vi "NKTP_API_UserEventExample.vi"() -> ()   [LabVIEW 2015]
doc: "This VI is a template that can be used when you want to make LabVIEW code that registers events from the NKTP driver as LabVIEW events in an event structure.\nPlease consult the \"NKTP_API_RegUserEvents.vi\" VI documentation for more information regarding using LabVIEW events with the NKTP driver."
uses:
  <instrlib>/NKTP_API/Public/Event/NKTP_API_RegisterDataType.ctl
  <instrlib>/NKTP_API/Private/NKTP_API_ParametersetType.ctl
  <instrlib>/NKTP_API/Public/Event/NKTP_API_DeviceStatusCallbackType.ctl
  <instrlib>/NKTP_API/Private/NKTP_API_DeviceCallbackStatusTypes.ctl
  <instrlib>/NKTP_API/Public/Event/NKTP_API_PortStatusCallbackType.ctl
  <instrlib>/NKTP_API/Private/NKTP_API_PortCallbackStatusTypes.ctl
  <instrlib>/NKTP_API/Public/Event/NKTP_API_RegisterStatusCallbackType.ctl
  <instrlib>/NKTP_API/Private/NKTP_API_RegisterCallbackStatusTypes.ctl
  <instrlib>/NKTP_API/Private/NKTP_API_RegisterDataTypes.ctl
  <instrlib>/NKTP_API/Private/NKTP_API_RegisterPriorityTypes.ctl
  <instrlib>/NKTP_API/NKTP_API.lvlib
panel:
  out "RegisterStatusCallbackData":T1={"portname"="", "devId"=0, "regId"=0, "status"=enum."RegSucces", "type"=enum."RegData_Array", "regDataLen"=0, "regData"=[]} {"regId" format="%.0x"}
  out "PortStatusCallbackData":T4={"portname"="", "status"=enum."PortStatusUnknown", "curScanAdr"=0, "maxScanAdr"=0, "foundType"=1}
  out "DeviceStatusCallbackData":T6
  in  "VISA Resource Name":refnum<visa-resource-name>
  out "RegisterData":T8
  out "error out":errorcluster
  in  "Close":bool
  in  "Open":bool
  in  "stop":bool
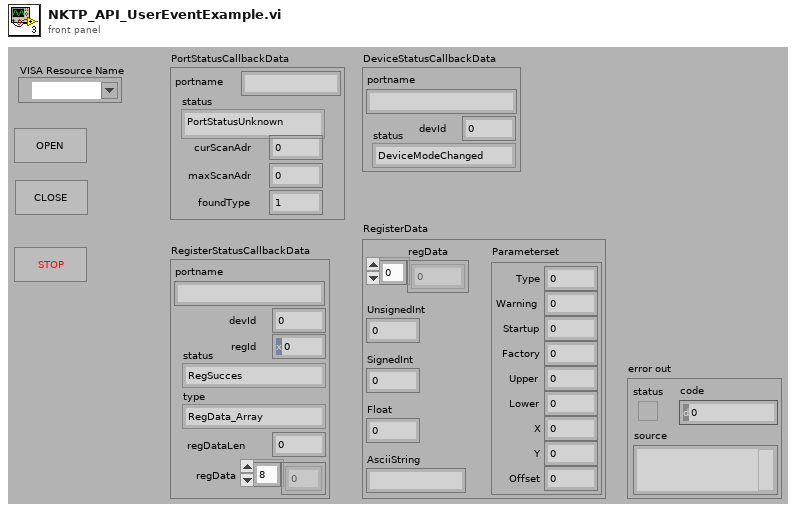
[diagram p1: front panel]
types:
  T1 = typedef "NKTP_API.lvlib/NKTP_API_RegisterStatusCallbackType.ctl" = cluster{"portname":string, "devId":u8, "regId":u8, "status":T2, "type":T3, "regDataLen":u8, "regData":u8[]}
  T2 = typedef "NKTP_API.lvlib/NKTP_API_RegisterCallbackStatusTypes.ctl" = enum8{"RegSucces", "RegBusy", "RegNacked", "RegCRCErr", "RegTimeout", "RegComError"}
  T3 = typedef "NKTP_API.lvlib/NKTP_API_RegisterDataTypes.ctl" = enum8{"RegData_Unknown", "RegData_Array", "RegData_U8", "RegData_S8", "RegData_U16", "RegData_S16", "RegData_U32", "RegData_S32", "RegData_F32", "RegData_U64", "RegData_S64", "RegData_F64", "RegData_Ascii", "RegData_Paramset"}
  T4 = typedef "NKTP_API.lvlib/NKTP_API_PortStatusCallbackType.ctl" = cluster{"portname":string, "status":T5, "curScanAdr":u8, "maxScanAdr":u8, "foundType":u16}
  T5 = typedef "NKTP_API.lvlib/NKTP_API_PortCallbackStatusTypes.ctl" = enum8{"PortStatusUnknown", "PortOpening", "PortOpened", "PortOpenFail", "PortScanStarted", "PortScanProgress", "PortScanDeviceFound", "PortScanEnded ", "PortClosing", "PortClosed", "PortReady"}
  T6 = typedef "NKTP_API.lvlib/NKTP_API_DeviceStatusCallbackType.ctl" = cluster{"portname":string, "devId":u8, "status":T7}
  T7 = typedef "NKTP_API.lvlib/NKTP_API_DeviceCallbackStatusTypes.ctl" = enum8{"DeviceModeChanged", "DeviceLiveChanged", "DeviceTypeChanged", "DevicePartNumberChanged", "DevicePCBVersionChanged", "DeviceStatusBitsChanged", "DeviceErrorCodeChanged", "DeviceBlVerChanged", "DeviceFwVerChanged", "DeviceModuleSerialChanged", "DevicePCBSerialChanged"}
  T8 = typedef "NKTP_API.lvlib/NKTP_API_RegisterDataType.ctl" = cluster{"regData":u8[], "UnsignedInt":u64, "SignedInt":i64, "Float":dbl, "AsciiString":string, "Parameterset":T9}
  T9 = typedef "NKTP_API.lvlib/NKTP_API_ParametersetType.ctl" = cluster{"Type":u8, "Warning":u8, "Startup":u16, "Factory":u16, "Upper":u16, "Lower":u16, "X":i16, "Y":i16, "Offset":i16}
  T10 = enum8{"Enabled", "Disabled", "Disabled and Grayed Out"}
  T11 = typedef "NKTP_API.lvlib/NKTP_API_RegisterPriorityTypes.ctl" = enum8{"RegPriority_Low", "RegPriority_High"}
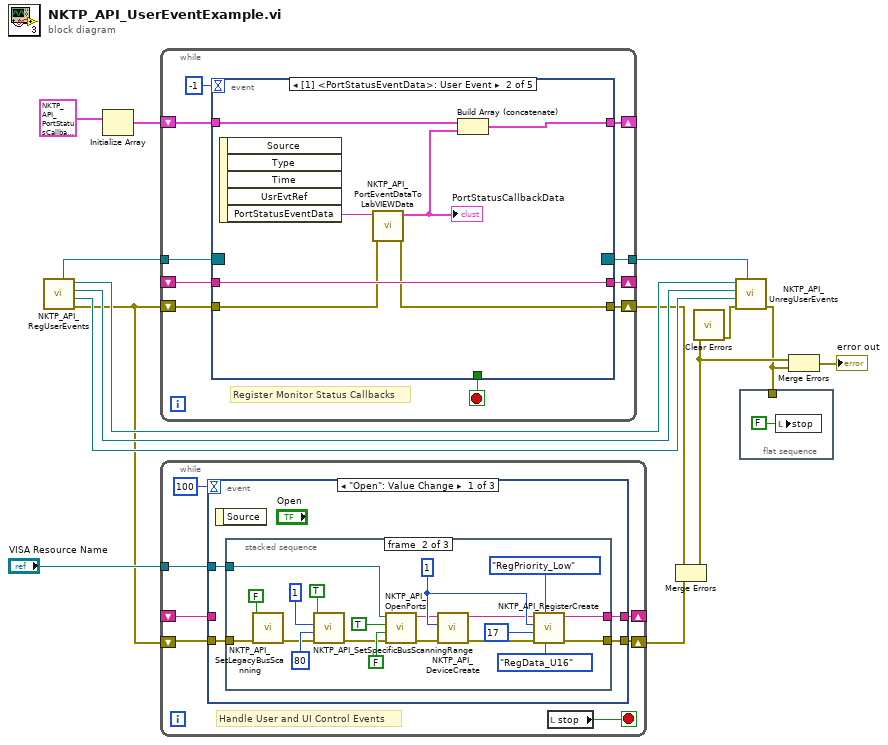
[diagram p0: block diagram]
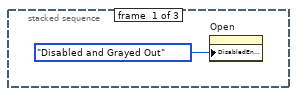
[diagram p2: hidden frame]
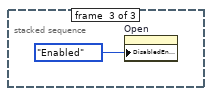
[diagram p3: hidden frame]
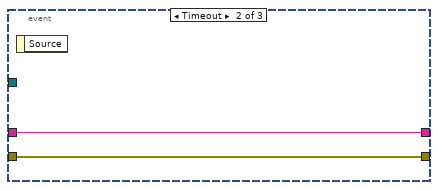
[diagram p4: hidden frame]
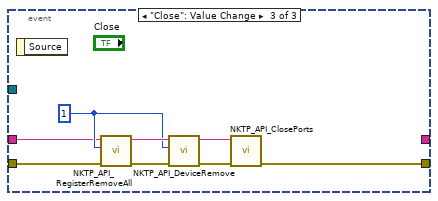
[diagram p5: hidden frame]
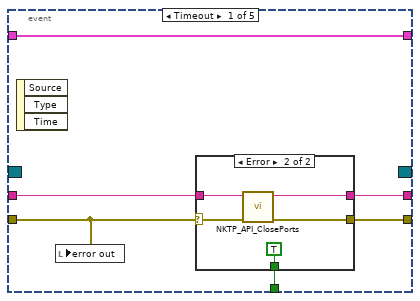
[diagram p6: hidden frame]
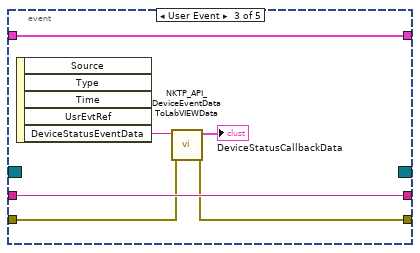
[diagram p8: hidden frame]
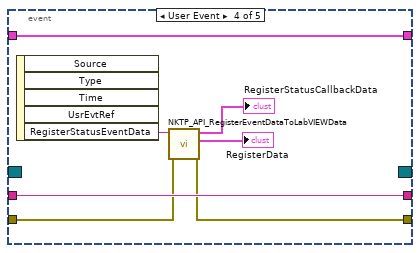
[diagram p9: hidden frame]
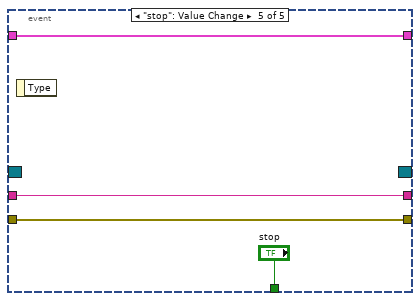
[diagram p10: hidden frame]
diagram:
  n1 = call <instrlib>:"NKTP_API_RegUserEvents.vi"() -> ("error out"=w9:errorcluster, "Register Status User Event"=w11:refnum<user-event>, "Device Status User Event"=w12:refnum<user-event>, "Port Status User Event"=w13:refnum<user-event>, "Event Registration Refnum"=w15:refnum<event-registration>)  [unwired: 7 in]
  n2 = Initialize Array(T4 {"portname"="COM1", "status"=enum."PortClosed", "curScanAdr"=0, "maxScanAdr"=0, "foundType"=0} ("PortStatusCallbackData")) -> (w7:T4[])  [unwired: 1 in]
  n3 = while {
    shift-right: [w23] -> _
    shift-left: _ -> [w22]
    shift-right: [w21] -> w5
    shift-left: w9 -> [w24]
    tunnel: [w19] -> w14
    tunnel: w15 -> [w18]
    shift-right: [w16] -> _
    shift-left: w7 -> [w17]
    stop <- w25 stop-if-true
    # "Register Monitor Status Callbacks"
    n4 = event shown="[1] <PortStatusEventData>: User Event" {
      selector: w18 -> [_ _ _ _ _]
      dyn-events: [_ _ _ _ _] -> w19
      timeout: -1 -> [_ _ _ _ _]
      tunnel: [w30 _ _ _ "stop"] -> w25
      tunnel: w24 -> [w27 w43 w48 w55 w60]
      tunnel: [w29 w45 w51 w58 w61] -> w23
      tunnel: w22 -> [w31 w45 w51 w58 w61]
      tunnel: [w28 w42 w47 w54 w60] -> w21
      tunnel: w17 -> [w26 w41 w46 w52 w59]
      tunnel: [w26 w39 w46 w52 w59] -> w16
      event Timeout {
        n5 = event-data() -> ()  [unwired: 1 in, 3 out]
        n6 = local write "error out"(w27) -> ()
        n7 = case shown="Error" w27 {
          selector: w27 -> [w32 w36]
          tunnel: w31 -> [w33 w37]
          tunnel: [_ TRUE] -> w30
          tunnel: [w33 w34] -> w29
          tunnel: [w32 w35] -> w28
          frame No Error {
          }
          frame Error {
            n8 = call <instrlib>:"NKTP_API_ClosePorts.vi"("error in"=w36, "portnames"=w37) -> ("error out"=w35:errorcluster, "portnames out"=w34:string)  [unwired: 8 in]
          }
        }
      }
      event User Event {
        n9 = event-data() -> ("PortStatusEventData"=w44:string)  [unwired: 1 in, 4 out]
        n10 = call <instrlib>:"NKTP_API_PortEventDataToLabVIEWData.vi"("error in"=w43, "PortStatusEventData"=w44) -> ("error out"=w42:errorcluster, "PortStatusCallbackData"=w40:T4)  [unwired: 8 in]
        "PortStatusCallbackData" <- w40
        n11 = Build Array (concatenate)(w41, w40) -> (w39:T4[])
      }
      event User Event {
        n12 = event-data() -> ("DeviceStatusEventData"=w50:string)  [unwired: 1 in, 4 out]
        n13 = call <instrlib>:"NKTP_API_DeviceEventDataToLabVIEWData.vi"("error in"=w48, "DeviceStatusEventData"=w50) -> ("error out"=w47:errorcluster, "DeviceStatusCallbackData"=→"DeviceStatusCallbackData":T6)  [unwired: 8 in]
      }
      event User Event {
        n14 = event-data() -> ("RegisterStatusEventData"=w57:string)  [unwired: 1 in, 4 out]
        n15 = call <instrlib>:"NKTP_API_RegisterEventDataToLabVIEWData.vi"("error in"=w55, "RegisterStatusEventData"=w57) -> ("error out"=w54:errorcluster, "RegisterData"=→"RegisterData":T8, "RegisterStatusCallbackData"=→"RegisterStatusCallbackData":T1)  [unwired: 7 in]
      }
      event "stop": Value Change {
        n16 = event-data() -> ()  [unwired: 1 in, 1 out]
      }
    }
  }
  n17 = while {
    tunnel: "VISA Resource Name" -> [w69]
    shift-right: [w67] -> w6
    shift-left: w9 -> [w68]
    shift-right: [w65] -> _
    shift-left: _ -> [w64]
    stop <- w63 stop-if-true
    # "Handle User and UI Control Events"
    n18 = event shown="[0] \"Open\": Value Change" {
      selector: _ -> [_ _ _]
      dyn-events: _ -> [_ _ _]
      timeout: 100 -> [_ _ _]
      tunnel: w69 -> [w73 _ _]
      tunnel: w68 -> [w71 w96 w100]
      tunnel: [w70 w96 w98] -> w67
      tunnel: [w72 w97 _] -> w65
      tunnel: w64 -> [_ w97 w99]
      event "Open": Value Change {
        n19 = event-data() -> ()  [unwired: 1 in, 1 out]
        n20 = stacked-sequence {
          tunnel: w73 -> [_ w86 _]
          tunnel: [_ w85 _] -> w72
          tunnel: w71 -> [_ w78 _]
          tunnel: [_ w75 _] -> w70
          frame #0 {
            n21 = property on="Open" class="Bool"("DisabledEnum"=T10."Disabled and Grayed Out" ("Disabled")) -> ()  [unwired: 2 in, 2 out]
          }
          frame #1 {
            w94 = u8 1 ("DevId")
            n22 = call <instrlib>:"NKTP_API_SetLegacyBusScanning.vi"("error in"=w78, "legacyMode"=FALSE) -> ("error out"=w77:errorcluster)  [unwired: 9 in]
            n23 = call <instrlib>:"NKTP_API_SetSpecificBusScanningRange.vi"("error in"=w77, "endAddress"=u8 80, "startAddress"=u8 1, "specificScanning"=TRUE) -> ("error out"=w83:errorcluster)  [unwired: 7 in]
            n24 = call <instrlib>:"NKTP_API_OpenPorts.vi"("error in"=w83, "liveMode"=FALSE ("LiveMode"), "autoMode"=TRUE, "portnames"=w86) -> ("error out"=w88:errorcluster, "portnames out"=w87:string)  [unwired: 6 in]
            n25 = call <instrlib>:"NKTP_API_DeviceCreate.vi"("error in"=w88, "devId"=w94, "portname"=w87) -> ("error out"=w92:errorcluster, "portname out"=w93:string)  [unwired: 7 in]
            n26 = call <instrlib>:"NKTP_API_RegisterCreate.vi"("dataType"=NKTP_API_RegisterDataTypes."RegData_U16" ("DataType"), "priority"=NKTP_API_RegisterPriorityTypes."RegPriority_Low" ("Priority"), "error in"=w92, "regId"=u8 17 ("RegId"), "devId"=w94, "portname"=w93) -> ("error out"=w75:errorcluster, "portname out"=w85:string)  [unwired: 4 in]
          }
          frame #2 {
            n27 = property on="Open" class="Bool"("DisabledEnum"=T10."Enabled" ("Disabled")) -> ()  [unwired: 2 in, 2 out]
          }
        }
      }
      event Timeout {
        n28 = event-data() -> ()  [unwired: 1 in, 1 out]
      }
      event "Close": Value Change {
        w101 = u8 1 ("DevId")
        n29 = event-data() -> ()  [unwired: 1 in, 1 out]
        n30 = call <instrlib>:"NKTP_API_RegisterRemoveAll.vi"("error in"=w100, "devId"=w101, "portname"=w99) -> ("error out"=w104:errorcluster, "portname out"=w105:string)  [unwired: 7 in]
        n31 = call <instrlib>:"NKTP_API_DeviceRemove.vi"("error in"=w104, "devId"=w101, "portname"=w105) -> ("error out"=w102:errorcluster, "portname out"=w103:string)  [unwired: 7 in]
        n32 = call <instrlib>:"NKTP_API_ClosePorts.vi"("error in"=w102, "portnames"=w103) -> ("error out"=w98:errorcluster)  [unwired: 8 in, 1 out]
      }
    }
    n33 = local read "stop"() -> (w63:bool)
  }
  n34 = Merge Errors(w5, w6) -> (w3:errorcluster)
  n35 = call <vilib>:"Clear Errors.vi"("error in (no error)"=w3) -> ("error out"=w4:errorcluster)  [unwired: 5 in, 1 out]
  n36 = call <instrlib>:"NKTP_API_UnregUserEvents.vi"("Event Registration Refnum"=w14, "error in"=w4, "Register Status User Event"=w11, "Device Status User Event"=w12, "Port Status User Event"=w13) -> ("error out"=w2:errorcluster)  [unwired: 6 in]
  n37 = flat-sequence {
    tunnel: w2 -> [_]
    frame #0 {
      n38 = local write "stop"(FALSE ("stop")) -> ()
    }
  }
  n39 = Merge Errors(w3, w2) -> (→"error out":errorcluster)
